vi "Set_Do_Array.vi"(8 "error in (no error)":errorcluster, 10 "DOs":bool[](array[boolean]), 11 "reference in":refnum<class "FPGA_Mock.lvclass">) -> (0 "error out":errorcluster, 3 "reference out":refnum<class "FPGA_Mock.lvclass">)   [LabVIEW 2019, in "FPGA_Mock.lvclass"]
uses:
  FPGA_Mock.lvclass
  FPGA_Mock.lvclass/FPGA_Mock.ctl
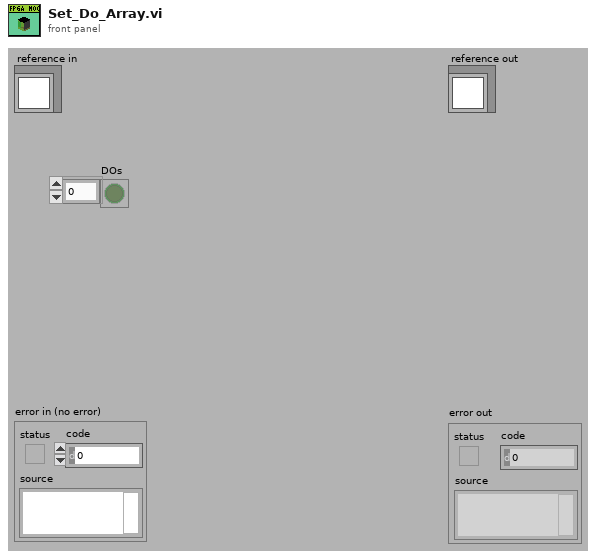
[diagram p1: front panel]
types:
  T1 = typedef "FPGA_Mock.lvclass/SharedData.ctl" = cluster{"DI":bool[], "DO":bool[], "AO":dbl[]}
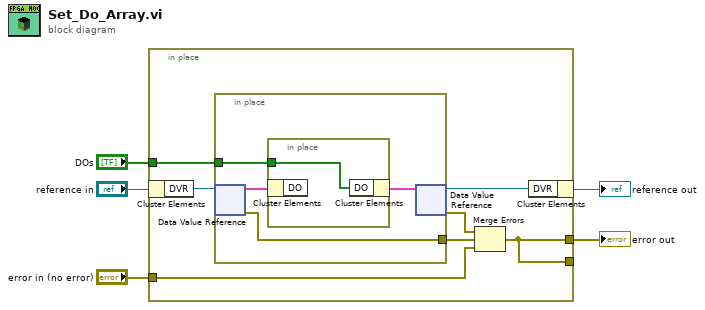
[diagram p0: block diagram]
diagram:
  n1 = in-place {
    in-place-border: "error in (no error)" -> [w8]
    in-place-border: [w6] -> _
    in-place-border: "DOs" -> [w7]
    in-place-border: [w6] -> w2
    n2 = in-place-cluster #1("reference in") -> ("DVR"=w12:refnum<data-value>)
    n3 = in-place {
      in-place-border: [w16] -> w10
      in-place-border: w7 -> [w13]
      n4 = in-place-dvr #2(w12) -> (w15:T1, w16:errorcluster)
      n5 = in-place {
        in-place-border: w13 -> [w17]
        n6 = in-place-cluster #3(w15) -> ()  [unwired: 1 out]
        n7 = in-place-cluster #3("DO"=w17) -> (w14:T1)
      }
      n8 = in-place-dvr #2(w14) -> (w11:refnum<data-value>, w9:errorcluster)
    }
    n9 = Merge Errors(w9, w10, w8) -> (w6:errorcluster)
    n10 = in-place-cluster #1("DVR"=w11) -> (→"reference out":refnum<class "FPGA_Mock.lvclass">)
  }
  "error out" <- w2
